vi "Simple State Machine.vi"() -> ()   [LabVIEW 2020]
doc: "Simple string based state machine with internal error handling.\n\n--------------------\n<Author>\n<Company>"
uses:
  Classes/Generic DAQ/Generic DAQ.lvclass
  Classes/DAQmx/DAQmx.lvclass
  C:/Users/juan_/Desktop/Lab it Studio/Public/Sesiones/Sesiones/Sesion [3] 24 Mar 2025/OOP Demo/Classes/Generic DAQ/Generic DAQ.lvclass
  Classes/34972A/34972A.lvclass
  <vilib>/ErrorRing/Error Ring.xnode
  <vilib>/Utility/error.llb/Error Cluster From Error Code.vi
panel:
  out "Voltage":dbl(graph)
  in  "Close":bool
  in  "Open":bool
  in  "Objects":enum16{"Sim", "DAQmx", "34972A"}(ring)
  in  "Stop":bool
  out "Error Out":errorcluster
  in  "Error In":errorcluster
  out "Status":string
  in  "Read Continously":bool
  in  "Read":bool
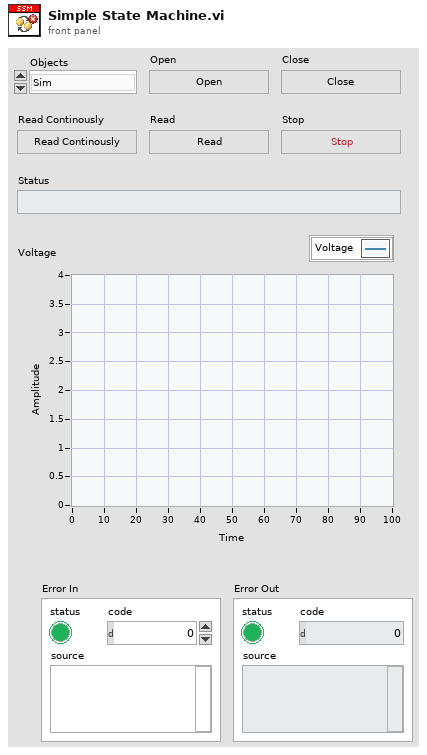
[diagram p1: front panel]
types:
  T1 = cluster{"Message":string, "DAQ":refnum<class "Generic DAQ.lvclass">, "Timeout":i32, "Voltage":dbl}
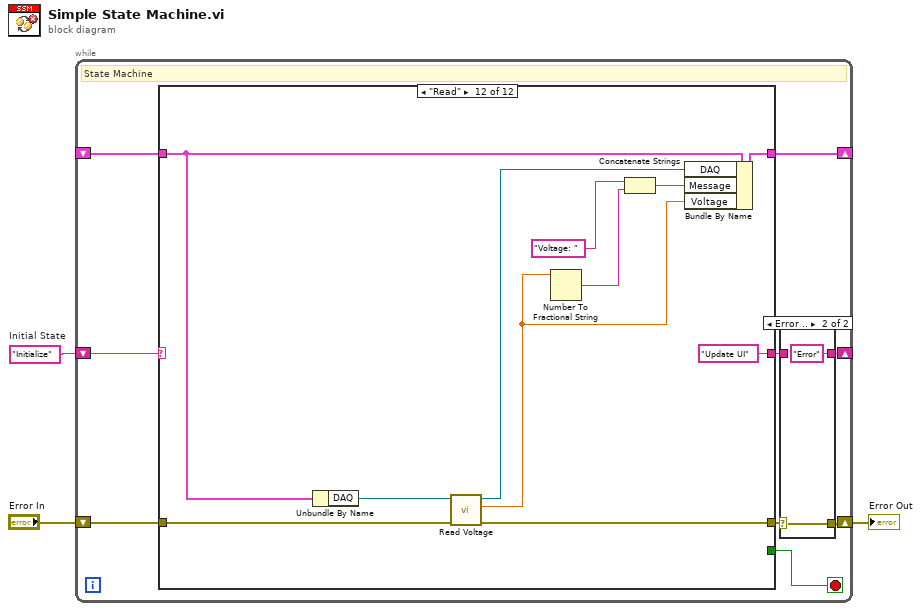
[diagram p0: block diagram]
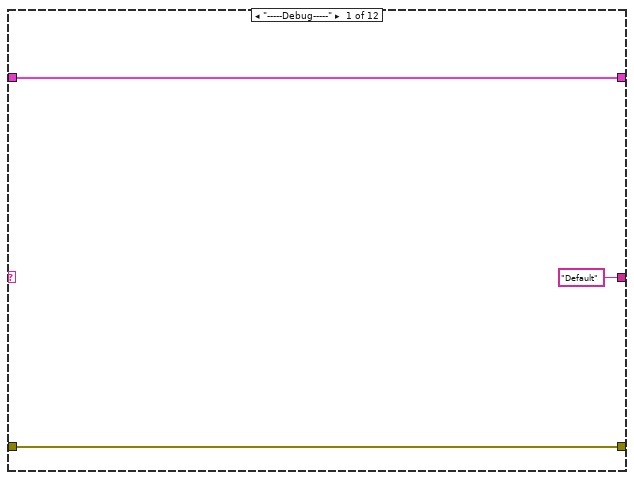
[diagram p3: hidden frame]
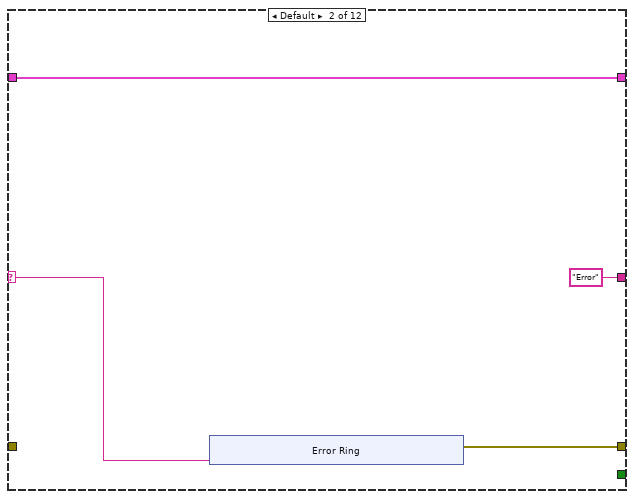
[diagram p4: hidden frame]
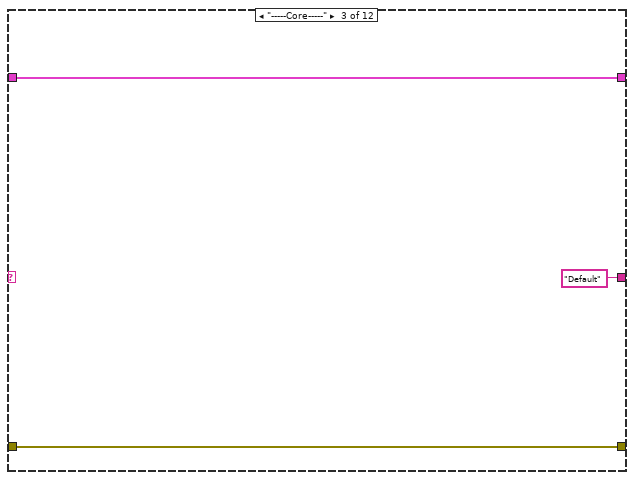
[diagram p5: hidden frame]
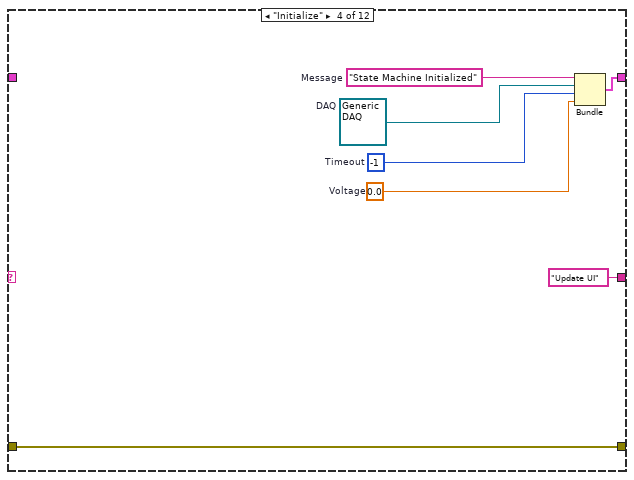
[diagram p6: hidden frame]
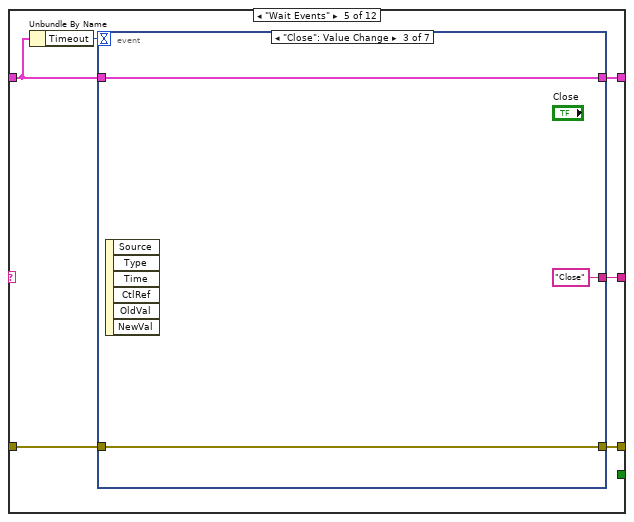
[diagram p7: hidden frame]
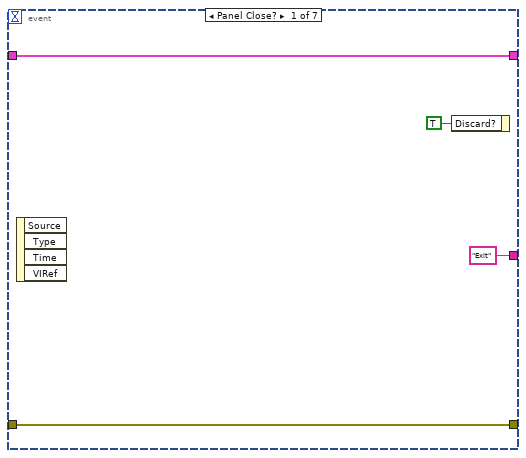
[diagram p8: hidden frame]
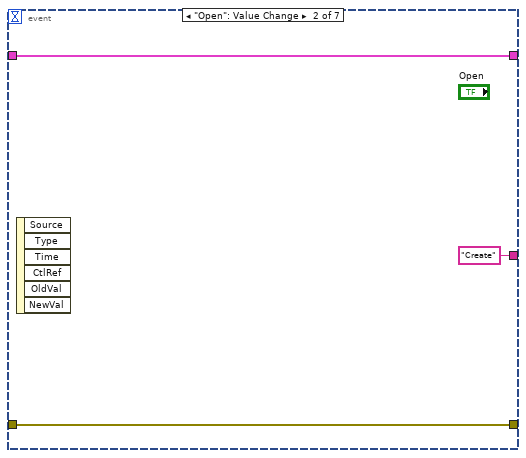
[diagram p9: hidden frame]
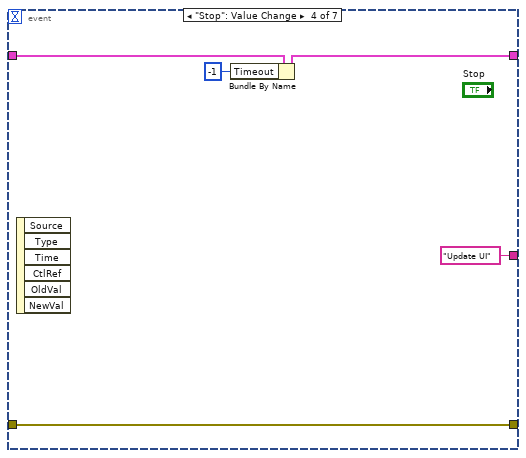
[diagram p10: hidden frame]
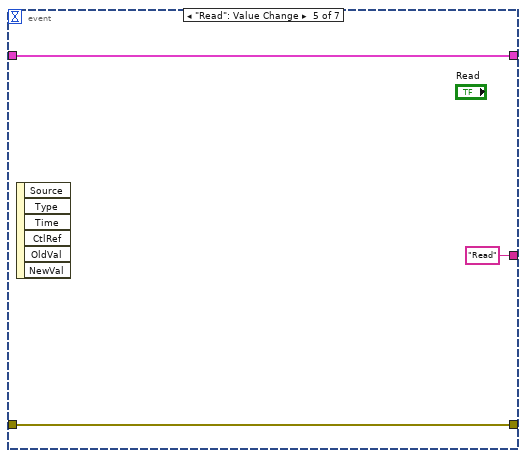
[diagram p11: hidden frame]
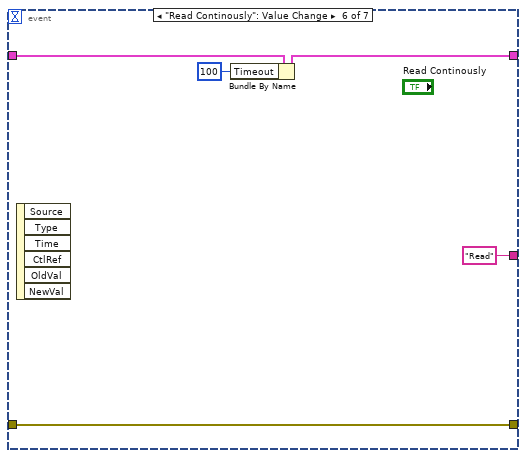
[diagram p12: hidden frame]
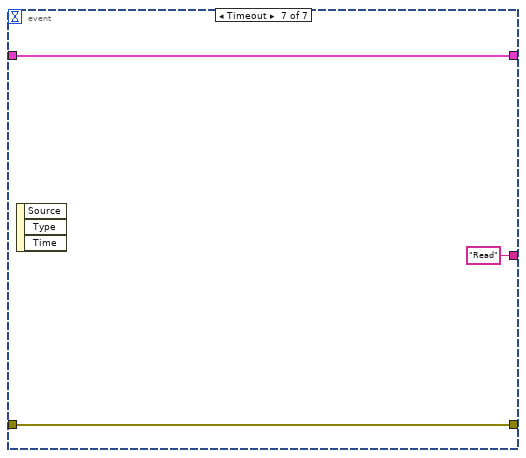
[diagram p13: hidden frame]
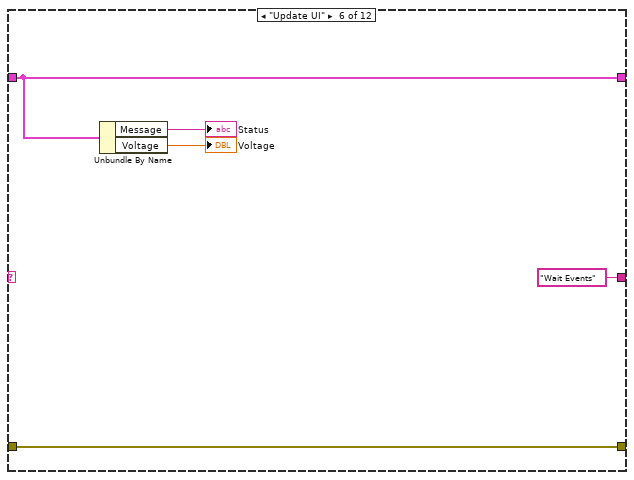
[diagram p14: hidden frame]
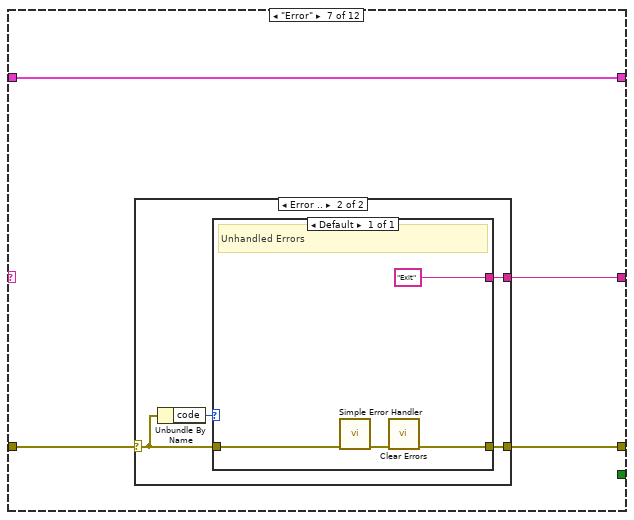
[diagram p15: hidden frame]
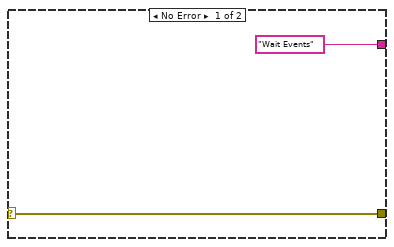
[diagram p16: hidden frame]
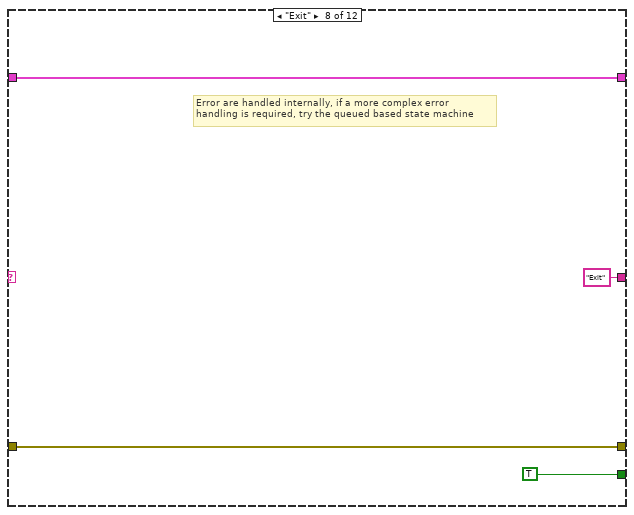
[diagram p17: hidden frame]
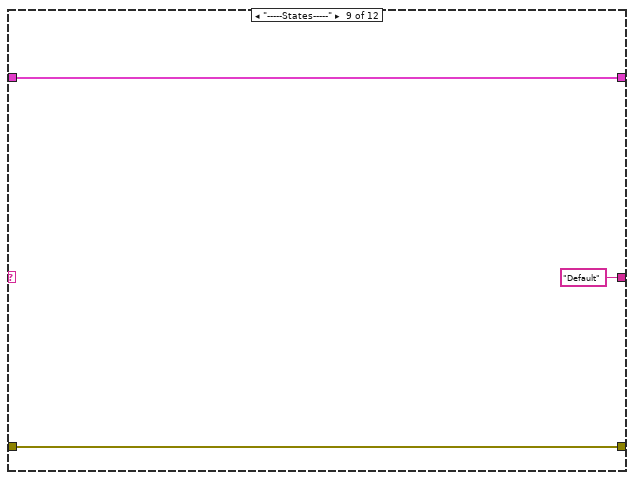
[diagram p18: hidden frame]
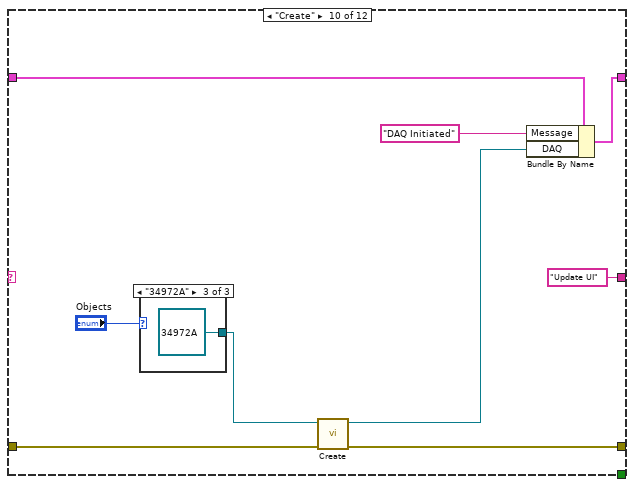
[diagram p19: hidden frame]
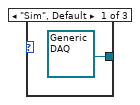
[diagram p20: hidden frame]
diagram:
  w1 = "Initialize"  # Initial State
  n1 = while {
    shift-right: [w4] -> _
    shift-left: w1 -> [w12]
    shift-right: [w10] -> _
    shift-left: _ -> [w11]
    shift-right: [w6] -> w3
    shift-left: "Error In" -> [w8]
    stop <- w9 stop-if-true
    # "State Machine"
    n2 = case shown="\"Read\"" w12 {
      selector: w12 -> [_ w21 _ _ _ _ _ _ _ _ _ _]
      tunnel: w8 -> [w19 _ w33 w40 w46 w77 w78 w95 w98 w102 w118 w129]
      tunnel: [w19 w22 w33 w40 w45 w77 w79 w95 w98 w103 w116 w128] -> w7
      tunnel: [_ _ _ _ _ _ _ TRUE _ _ _ _] -> w9
      tunnel: ["Default" ("State") "Error" ("Next State") "Default" ("Next State") "Update UI" ("Next State") w44 "Wait Events" ("State") w80 "Exit" ("State") "Default" ("State") "Update UI" ("State") "Update UI" ("State") "Update UI" ("State")] -> w5
      tunnel: w11 -> [w18 w23 w32 _ w42 w76 w81 w92 w97 w104 w115 w127]
      tunnel: [w18 w23 w32 w38 w43 w76 w81 w92 w97 w106 w113 w125] -> w10
      frame "-----Debug-----" {
        # "State used for organization purposes."
      }
      frame Default {
        # "Default state used to debug undeclared states."
        n3 = xnode "Error Ring"("parameter 0"=w21) -> ("error out"=w22:errorcluster)
      }
      frame "-----Core-----" {
        # "State used for organization purposes."
      }
      frame "Initialize" {
        w34 = 0.0  # Voltage
        w35 = -1  # Timeout
        w36 = refnum<class "Generic DAQ.lvclass"> refnum  # DAQ
        w39 = "State Machine Initialized"  # Message
        # "Initialize the state machine."
        n4 = Bundle("Message"=w39, "DAQ"=w36, "Timeout"=w35, "Voltage"=w34) -> (w38:T1)  [unwired: 1 in]
      }
      frame "Wait Events" {
        # "Wait for Events"
        n5 = Unbundle By Name(w42) -> ("Timeout"=w41:i32)
        n6 = event shown="[2] \"Close\": Value Change" {
          selector: _ -> [_ _ _ _ _ _ _]
          dyn-events: _ -> [_ _ _ _ _ _ _]
          timeout: w41 -> [_ _ _ _ _ _ _]
          tunnel: w46 -> [w47 w53 w56 w61 w63 w69 w72]
          tunnel: [w47 w53 w56 w61 w63 w69 w72] -> w45
          tunnel: ["Exit" ("State") "Create" ("State") "Close" ("State") "Update UI" ("State") "Read" ("State") "Read" ("State") "Read" ("State")] -> w44
          tunnel: w42 -> [w48 w52 w55 w60 w62 w67 w71]
          tunnel: [w48 w52 w55 w58 w62 w66 w71] -> w43
          event Panel Close? {
            # "Stop button value change event."
            n7 = event-data() -> ()  [unwired: 1 in, 4 out]
            n8 = event-data("Discard?"=TRUE) -> ()  [unwired: 1 in, 1 out]
          }
          event "Open": Value Change {
            n9 = event-data() -> ()  [unwired: 1 in, 6 out]
          }
          event "Close": Value Change {
            n10 = event-data() -> ()  [unwired: 1 in, 6 out]
          }
          event "Stop": Value Change {
            n11 = event-data() -> ()  [unwired: 1 in, 6 out]
            n12 = Bundle By Name(cluster=w60, "Timeout"=-1) -> (w58:T1)
          }
          event "Read": Value Change {
            # "Ultimate Answer button value change event."
            n13 = event-data() -> ()  [unwired: 1 in, 6 out]
          }
          event "Read Continously": Value Change {
            # "Ultimate Question button value change event."
            n14 = event-data() -> ()  [unwired: 1 in, 6 out]
            n15 = Bundle By Name(cluster=w67, "Timeout"=100) -> (w66:T1)
          }
          event Timeout {
            n16 = event-data() -> ()  [unwired: 1 in, 3 out]
          }
        }
      }
      frame "Update UI" {
        # "Update User Interface"
        n17 = Unbundle By Name(w76) -> ("Message"=→"Status":string, "Voltage"=→"Voltage":dbl)
      }
      frame "Error" {
        n18 = case shown="Error .." w78 {
          selector: w78 -> [w83 w86]
          tunnel: [w83 w85] -> w79
          tunnel: ["Wait Events" ("Next State") w84] -> w80
          frame No Error {
          }
          frame Error {
            n19 = Unbundle By Name(w86) -> ("code"=w87:i32)
            n20 = case shown="Default" w87 {
              tunnel: w86 -> [w91]
              tunnel: [w89] -> w85
              tunnel: ["Exit" ("Next State")] -> w84
              frame Default {
                # "Unhandled Errors"
                n21 = call <vilib>:"Simple Error Handler.vi"("error in (no error)"=w91) -> ("error out"=w90:errorcluster)  [unwired: 4 in, 4 out]
                n22 = call <vilib>:"Clear Errors.vi"("error in (no error)"=w90) -> ("error out"=w89:errorcluster)  [unwired: 5 in, 1 out]
              }
            }
          }
        }
      }
      frame "Exit" {
        # "Error are handled internally, if a more complex error\nhandling is required, try the queued based state machine"
        # "Exit the State Machine"
      }
      frame "-----States-----" {
        # "State used for organization purposes."
      }
      frame "Create" {
        # "Ultimate Answer Event"
        n23 = case shown="\"34972A\"" "Objects" {
          tunnel: [refnum<class "Generic DAQ.lvclass"> refnum ("Generic DAQ.lvclass") refnum<class "DAQmx.lvclass"> refnum ("DAQmx.lvclass") refnum<class "34972A.lvclass"> refnum ("34972A.lvclass")] -> w99
          frame "Sim", Default {
          }
          frame "DAQmx" {
          }
          frame "34972A" {
          }
        }
        n24 = call-dynamic "Create.vi"("error in (no error)"=w102, "Generic DAQ in"=w99) -> ("error out"=w103:errorcluster, "Generic DAQ out"=w101:refnum<class "Generic DAQ.lvclass">)  [unwired: 8 in]
        n25 = Bundle By Name(cluster=w104, "Message"="DAQ Initiated", "DAQ"=w101) -> (w106:T1)
      }
      frame "Close" {
        # "Ultimate Question Event"
        n26 = Unbundle By Name(w115) -> ("DAQ"=w114:refnum<class "Generic DAQ.lvclass">)
        n27 = call-dynamic "Close.vi"("error in (no error)"=w118, "Generic DAQ in"=w114) -> ("error out"=w116:errorcluster, "Generic DAQ out"=w112:refnum<class "Generic DAQ.lvclass">)  [unwired: 8 in]
        n28 = Bundle By Name(cluster=w115, "Message"="DAQ Closed", "DAQ"=w112) -> (w113:T1)
      }
      frame "Read" {
        n29 = Unbundle By Name(w127) -> ("DAQ"=w126:refnum<class "Generic DAQ.lvclass">)
        n30 = call-dynamic "Read Voltage.vi"("error in (no error)"=w129, "Generic DAQ in"=w126) -> ("error out"=w128:errorcluster, "Voltage"=w119:dbl, "Generic DAQ out"=w124:refnum<class "Generic DAQ.lvclass">)  [unwired: 7 in]
        n31 = Number To Fractional String(number=w119) -> (F-format string=w122:string)  [unwired: 3 in]
        n32 = Concatenate Strings("Voltage: " ("string"), w122) -> (w120:string)
        n33 = Bundle By Name(cluster=w127, "DAQ"=w124, "Message"=w120, "Voltage"=w119) -> (w125:T1)
      }
    }
    n34 = case shown="Error .." w7 {
      selector: w7 -> [w14 w16]
      tunnel: [w14 w16] -> w6
      tunnel: w5 -> [w13 _]
      tunnel: [w13 "Error" ("State")] -> w4
      frame No Error {
      }
      frame Error {
      }
    }
  }
  "Error Out" <- w3
